vi "Project 1.vi"() -> ()   [LabVIEW 2024]
panel:
  in  "stop":bool
  out "Green":bool
  out "Blue":bool
  out "Red":bool
  out "H":dbl(slide) scale=0.0..10.0
  out "Rs":dbl(slide) scale=0.0..10.0
  out "vP":dbl(slide) scale=0.0..10.0
  out "vDiff":dbl(slide) scale=0.0..10.0
  out "\"SCC Volts":dbl format="%_3f"
  out "AD2 Input":i16 format="%04x"
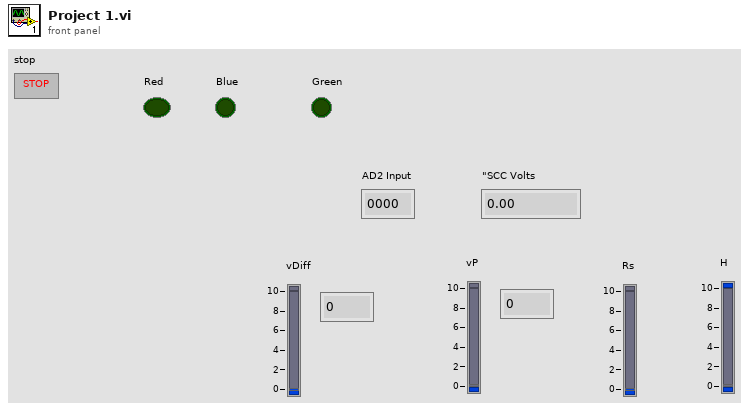
[diagram p1: front panel]
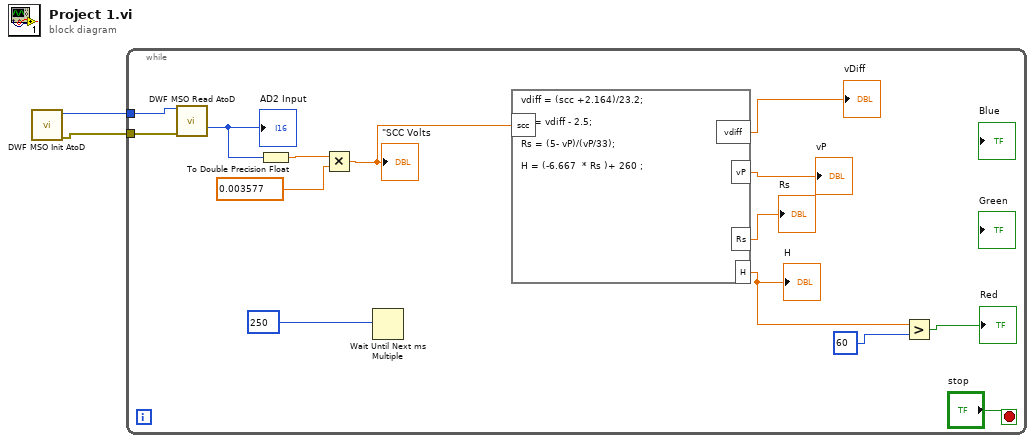
[diagram p0: block diagram]
diagram:
  n1 = call "DWF MSO Init AtoD.vi"() -> ("Error Out"=w1:errorcluster, "Instrument Handle Out"=w2:u32)  [unwired: 10 in]
  n2 = while {
    tunnel: w2 -> [w6]
    tunnel: w1 -> [w5]
    stop <- "stop" stop-if-true
    n3 = call "DWF MSO Read AtoD.vi"("Instrument Handle In AtoD"=w6, "Error In"=w5) -> ("AtoD"=w4:i16)  [unwired: 12 in, 1 out]
    "AD2 Input" <- w4
    n4 = To Double Precision Float(number=w4) -> (double precision float=w15:dbl)
    n5 = Multiply(x=w15, y=0.003577) -> (x*y=w13:dbl)
    "\"SCC Volts" <- w13
    n6 = Wait Until Next ms Multiple(millisecond multiple=250) -> ()  [unwired: 1 out]
    n7 = formula code="vdiff = (scc +2.164)/23.2;\n\nvP = vdiff - 2.5;\n\nRs = (5- vP)/(vP/33);\n\nH = (-6.667  * Rs )+ 260 ;"("scc"=w13) -> ("vdiff"=→"vDiff":dbl, "vP"=→"vP":dbl, "Rs"=→"Rs":dbl, "H"=w10:dbl)
    "H" <- w10
    n8 = Greater?(x=w10, y=60) -> (0:→"Red":bool)
  }
